vi "runtest Check Instruments for Valid Configuration.vi"(6 "TestStation IP (\"\")":string, 8 "error in (no error)":errorcluster, 9 "Required Instruments In":T2[](array[typedef]), 11 "Connection Refnum":T1) -> (0 "error out":errorcluster, 1 "Required Instruments Out":T2[](array[typedef]), 3 "Connection Refnum":T1)   [LabVIEW 2011]
uses:
  server/database/Stations/Instruments/Instrument Record.ctl
  Summitek EXT/ODBC/SQL Controls/Connection Refnum.ctl
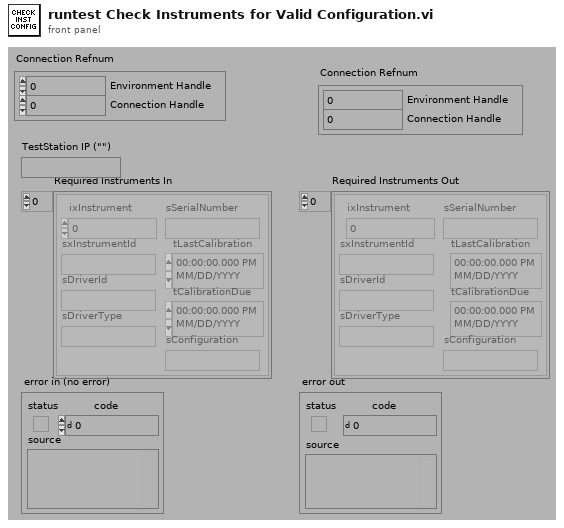
[diagram p1: front panel]
types:
  T1 = typedef "Connection Refnum.ctl" = cluster{"Environment Handle":i32, "Connection Handle":i32}
  T2 = typedef "Instrument Record.ctl" = cluster{"ixInstrument":i32, "sxInstrumentId":string, "sDriverId":string, "sDriverType":string, "sSerialNumber":string, "tLastCalibration":timestamp, "tCalibrationDue":timestamp, "sConfiguration":string}
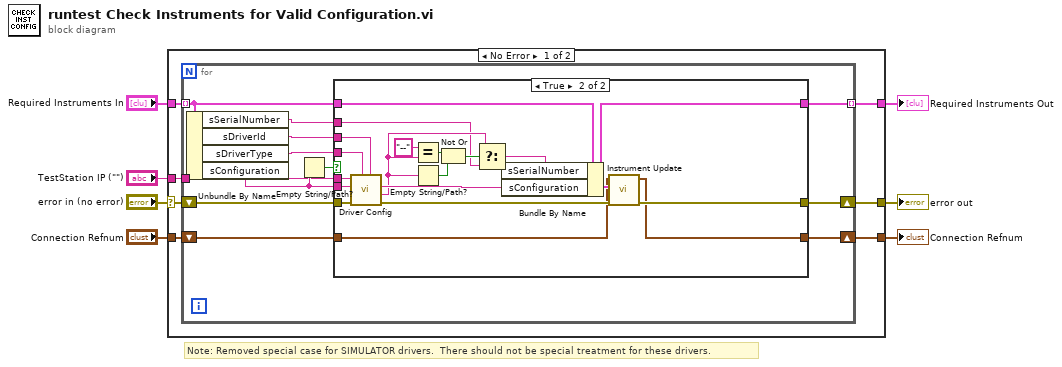
[diagram p0: block diagram]
diagram:
  # "Note: Removed special case for SIMULATOR drivers.  There should not be special treatment for these drivers."
  n1 = case shown="No Error" "error in (no error)" {
    selector: "error in (no error)" -> [w14 w51]
    tunnel: "Required Instruments In" -> [w12 w50]
    tunnel: [w13 w51] -> w5
    tunnel: [w11 w50] -> w4
    tunnel: "TestStation IP (\"\")" -> [w10 _]
    tunnel: "Connection Refnum" -> [w9 w49]
    tunnel: [w8 w49] -> w1
    frame No Error {
      n2 = for {
        shift-right: [w24] -> w13
        shift-left: w14 -> [w26]
        tunnel: w12 -> [w25] mode=indexing
        tunnel: [w23] -> w11 mode=indexing
        tunnel: w10 -> [w19]
        shift-right: [w16] -> w8
        shift-left: w9 -> [w17]
        n3 = Unbundle By Name(w25) -> ("sSerialNumber"=w20:string, "sDriverId"=w18:string, "sDriverType"=w22:string, "sConfiguration"=w21:string)
        n4 = Empty String/Path?(string/path=w21) -> (empty?=w15:bool)
        n5 = case shown="True" w15 {
          tunnel: w26 -> [w29 w48]
          tunnel: w25 -> [w28 w47]
          tunnel: [w29 w32] -> w24
          tunnel: [w28 w34] -> w23
          tunnel: w18 -> [_ w45]
          tunnel: w22 -> [_ w44]
          tunnel: w21 -> [_ w43]
          tunnel: w20 -> [_ w37]
          tunnel: w19 -> [_ w35]
          tunnel: w17 -> [w27 w31]
          tunnel: [w27 w30] -> w16
          frame False {
          }
          frame True {
            n6 = call "Driver Config.vi"("DriverID (\"\")"=w45, "DriverType (\"\")"=w44, "error in (no error)"=w48, "Configuration In (Empty)"=w43, "TestStation Client (\"\")"=w35) -> ("error out"=w33:errorcluster, "Serial Number"=w38:string, "Configuration Out"=w46:string)  [unwired: 1 in, 3 out]
            n7 = Equal?(x="--" ("y"), y=w38) -> (x = y?=w40:bool)
            n8 = Empty String/Path?(string/path=w38) -> (empty?=w41:bool)
            n9 = Not Or(1:w41, 2:w40) -> (0:w39:bool)
            n10 = Select(t=w38, s=w39, f=w37) -> (s? t:f=w36:string)
            n11 = Bundle By Name(cluster=w47, "sSerialNumber"=w36, "sConfiguration"=w46) -> (w34:T2)
            n12 = call "Instrument Update.vi"("error in (no error)"=w33, "Instrument Record"=w34, "Connection Refnum"=w31) -> ("error out"=w32:errorcluster, "Connection Refnum"=w30:T1)  [unwired: 7 out]
          }
        }
      }
    }
    frame Error {
    }
  }
  "error out" <- w5
  "Required Instruments Out" <- w4
  "Connection Refnum" <- w1
